vi "String Indicator.vi"(10 "String Indicator":string, 11 "Hello World Event in":refnum<class "Hello World Event.lvclass">) -> (3 "Hello World Event out":refnum<class "Hello World Event.lvclass">)   [LabVIEW 2021, in "Hello World Event.lvlib" / "Hello World Event.lvclass"]
uses:
  Hello World Event.lvclass
  Hello World Event.lvclass/Hello World Event.ctl
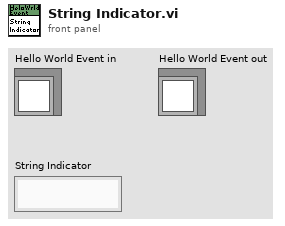
[diagram p1: front panel]
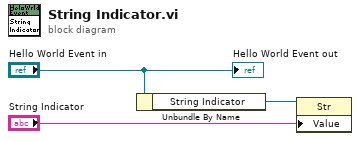
[diagram p0: block diagram]
diagram:
  n1 = Unbundle By Name("Hello World Event in") -> ("String Indicator"=w3:refnum<vi>)
  n2 = property class="Str"(reference=w3, "Value"="String Indicator") -> ()  [unwired: 1 in, 2 out]
  "Hello World Event out" <- "Hello World Event in"
